vi "StartAllAbsoluteMove.vi"(8 "error in (no error)":errorcluster, 9 "Positions, steps":T1, 10 "Current Z pos., mm":dbl, 11 "VXMMotionManager in":refnum<class "VXMMotionManager.lvclass">) -> (0 "error out":errorcluster, 3 "VXMMotionManager out":refnum<class "VXMMotionManager.lvclass">)   [LabVIEW 2018, in "VXMMotionManager.lvclass"]
doc: "put positions in the X,Y,Z,T target position and sets state to start.\nSequence Motion.vi should be called next, repeatedly, to finish the sequence of motion on all axes.\n\nMove Z up a little before every move. We used to move Z to home, but cutyomer requested not so far. All I can do is move Z up a little relative to it's current postion. I think this is better than moving Z up relative to the new Z target position. the only other soln. would be to put a Z Absolute Safe Position in the ini file, like a \"Home-2\" absolute position."
uses:
  VXMMotionManager.lvclass
  MoveAllAbsoluteStates.ctl
  Position.ctl
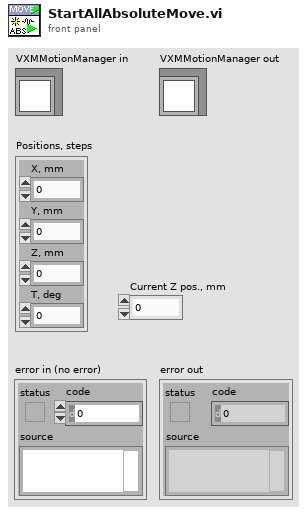
[diagram p1: front panel]
types:
  T1 = typedef "Position.ctl" = cluster{"X, mm":dbl, "Y, mm":dbl, "Z, mm":dbl, "T, deg":dbl}
  T2 = typedef "VXMMotionManager.lvclass/MoveAllAbsoluteStates.ctl" = enum16{"start next move", "wait motion end"}
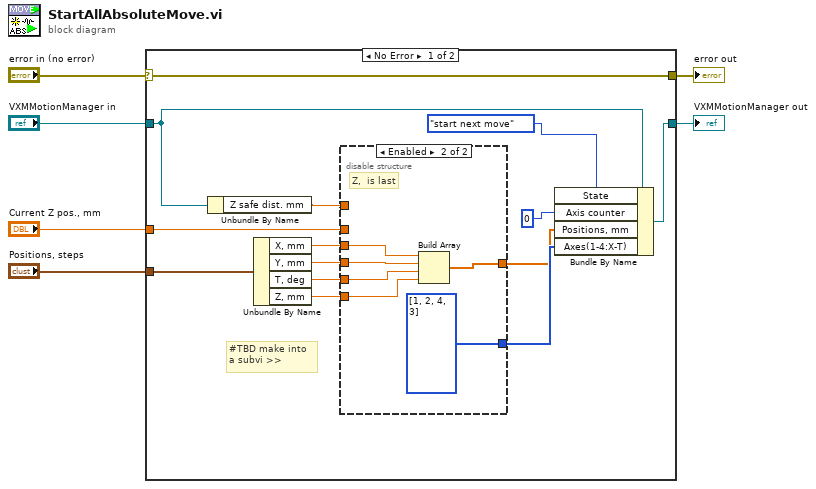
[diagram p0: block diagram]
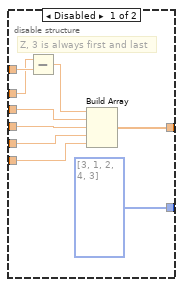
[diagram p2: hidden frame]
diagram:
  n1 = case shown="No Error" "error in (no error)" {
    selector: "error in (no error)" -> [w20 w37]
    tunnel: [w20 w37] -> w5
    tunnel: [w18 w36] -> w3
    tunnel: "VXMMotionManager in" -> [w13 w36]
    tunnel: "Positions, steps" -> [w17 _]
    tunnel: "Current Z pos., mm" -> [w7 _]
    frame No Error {
      # "#TBD make into\na subvi >>"
      n2 = Unbundle By Name(w13) -> ("Z safe dist. mm"=w9:dbl)
      n3 = Unbundle By Name(w17) -> ("X, mm"=w12:dbl, "Y, mm"=w11:dbl, "T, deg"=w10:dbl, "Z, mm"=w8:dbl)
      n4 = disable-structure shown="Enabled" {
        disable-tunnel: [i32[] [3, 1, 2, 4, 3] ("Axes(1-4:X-R)") i32[] [1, 2, 4, 3] ("Axes(1-4:X-R)")] -> w16
        disable-tunnel: [w28 w34] -> w14
        disable-tunnel: w12 -> [w27 w33]
        disable-tunnel: w11 -> [w26 w32]
        disable-tunnel: w10 -> [w25 w31]
        disable-tunnel: w9 -> [w24 _]
        disable-tunnel: w8 -> [w22 w30]
        disable-tunnel: w7 -> [w21 _]
        frame Disabled {
          # "Z, 3 is always first and last"
          n5 = Subtract(x=w21, y=w24) -> (x-y=w23:dbl)
          n6 = Build Array(w23, w27, w26, w25, w22) -> (w28:dbl[])
        }
        frame Enabled {
          # "Z,  is last"
          n7 = Build Array(w33, w32, w31, w30) -> (w34:dbl[])
        }
      }
      n8 = Bundle By Name(cluster=w13, "State"=MoveAllAbsoluteStates."start next move", "Axis counter"=0 ("Axis (0-3)"), "Positions, mm"=w14, "Axes(1-4:X-T)"=w16) -> (w18:refnum<class "VXMMotionManager.lvclass">)
    }
    frame Error {
    }
  }
  "error out" <- w5
  "VXMMotionManager out" <- w3
